vi "G4BaseTemplate_Singleton_5x6x5_SetProperty.vi"(7 "Property":dbl, 11 "error in (no error)":errorcluster) -> (15 "error out":errorcluster)   [LabVIEW 2014]
uses:
  <resource>/Framework/Providers/Open_GDS/ClassProviders/Provider_EndevoGOOP400/Templates/G4BaseTemplate_Singleton_5x6x5/G4BaseTemplate_Singleton_5x6x5.lvclass
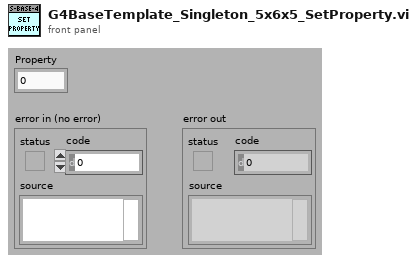
[diagram p1: front panel]
types:
  T1 = typedef "G4BaseTemplate_Singleton_5x6x5.lvclass/ObjectAttributes.ctl" = cluster{"Attribute1":dbl}
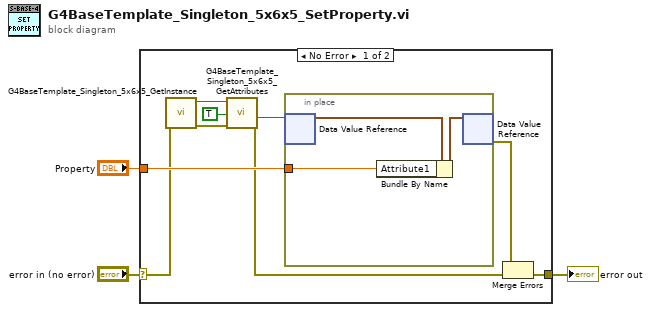
[diagram p0: block diagram]
diagram:
  n1 = case shown="No Error" "error in (no error)" {
    selector: "error in (no error)" -> [w6 w16]
    tunnel: [w10 w16] -> w2
    tunnel: "Property" -> [w12 _]
    frame No Error {
      n2 = call <resource>:"G4BaseTemplate_Singleton_5x6x5_GetInstance.vi"("error in (no error)"=w6) -> ("error out"=w8:errorcluster, "reference out"=w7:refnum<class "G4BaseTemplate_Singleton_5x6x5.lvclass">)  [unwired: 6 in, 3 out]
      n3 = call <resource>:"G4BaseTemplate_Singleton_5x6x5_GetAttributes.vi"("error in (no error)"=w8, "OnlyGetDvrReference(False)"=TRUE, "reference in"=w7) -> ("error out"=w9:errorcluster, "DataRef"=w5:refnum<data-value>)  [unwired: 5 in, 2 out]
      n4 = in-place {
        in-place-border: w12 -> [w15]
        n5 = in-place-dvr #1(w5) -> (w14:T1)  [unwired: 1 out]
        n6 = Bundle By Name(cluster=w14, "Attribute1"=w15) -> (w13:T1)
        n7 = in-place-dvr #1(w13) -> (w11:errorcluster)  [unwired: 1 out]
      }
      n8 = Merge Errors(w11, w9) -> (w10:errorcluster)
    }
    frame Error {
    }
  }
  "error out" <- w2
